vi "baseStation.vi"() -> ()   [LabVIEW 2012]
uses:
  <vilib>/Instr/_visa.llb/VISA Configure Serial Port (Instr).vi
panel:
  out "Cal Constants":u8[](array[numeric])
  in  "Auto Lock":bool
  in  "search mode":bool
  out "Found Radios":u8[](array[numeric])
  in  "shared variable refnum":refnum<k21>
  out "Humidity":dbl
  out "Temperature":dbl
  out "Pressure":dbl
  out "Magnetometer":dbl[](array[numeric])
  out "Gyro":dbl[](array[numeric])
  out "Acceleration":dbl[](array[numeric])
  out "Cal constants":string
  in  "State":T1(ring)
  out "output cluster":errorcluster
  in  "Stop Button":bool
  in  "Radio Address":dbl
  in  "Search for radio":bool
  in  "Com port":refnum<visa-resource-name>
  # "Active"
  # "Passive"
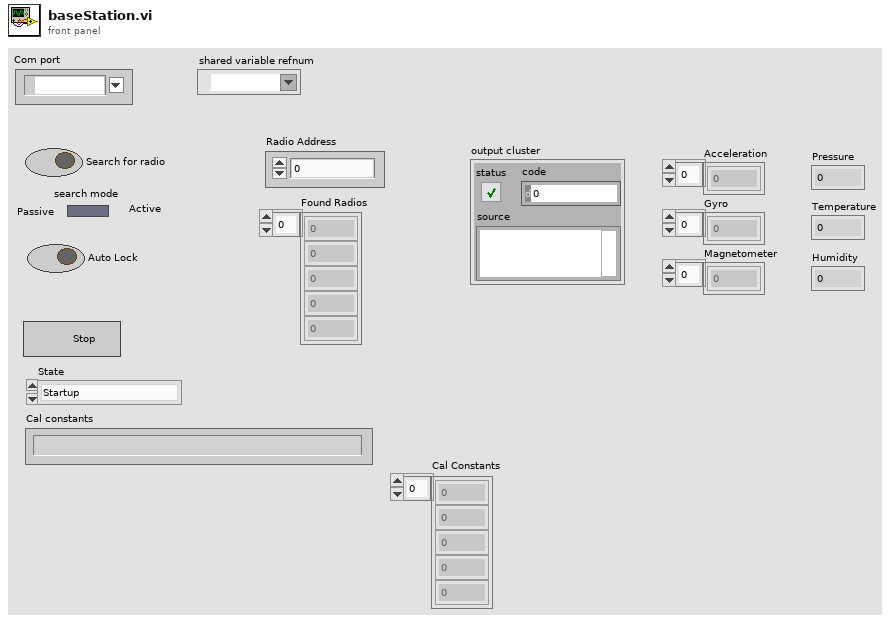
[diagram p1: front panel]
types:
  T1 = enum16{"Startup", "Start Search", "Active Search", "Start Single", "Run Single", "Shutdown", "Change Address"}
  T2 = cluster{"Acceleration":dbl[], "Gyro":dbl[], "Magnetometer":dbl[], "Temperature":dbl, "Pressure":dbl, "Humidity":dbl}
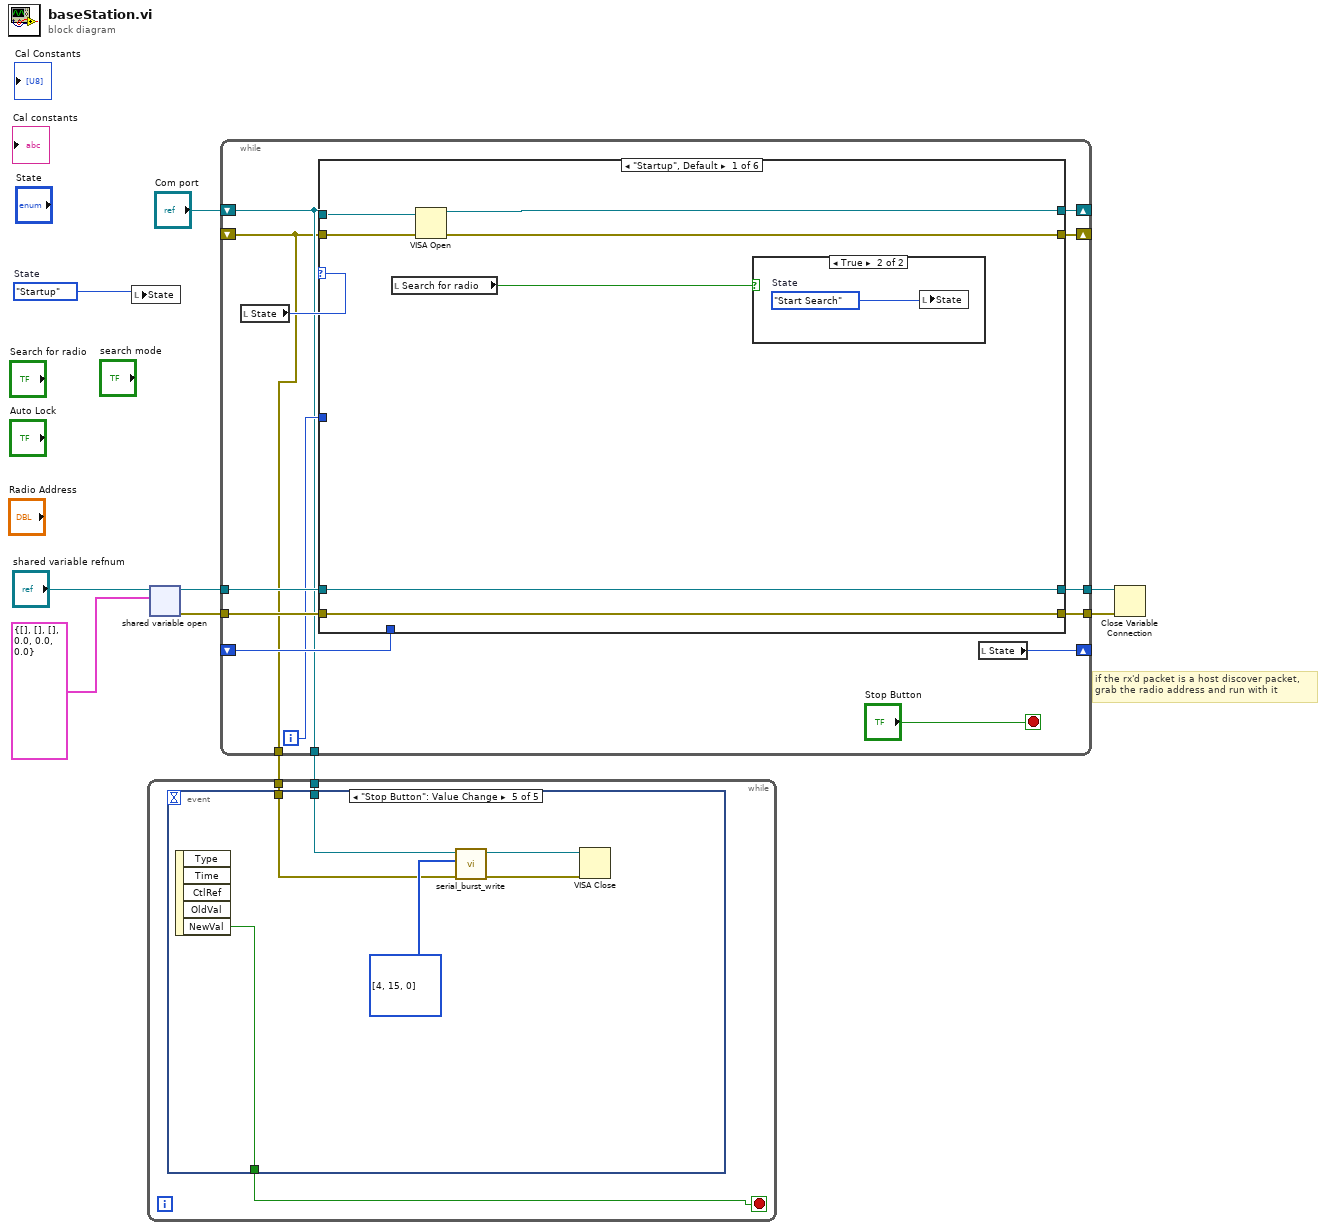
[diagram p0: block diagram]
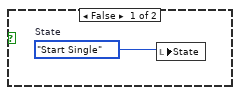
[diagram p2: hidden frame]
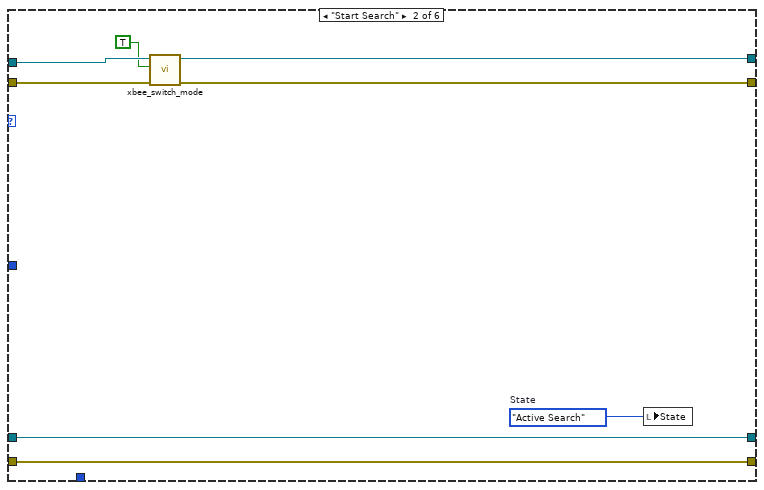
[diagram p3: hidden frame]
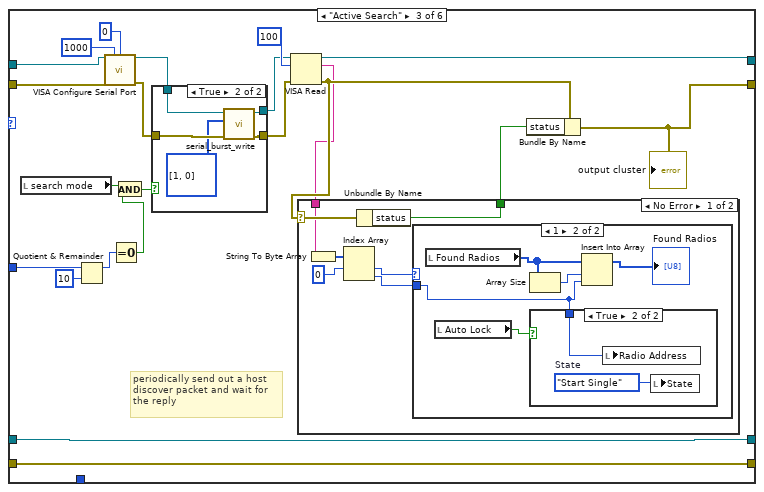
[diagram p4: hidden frame]
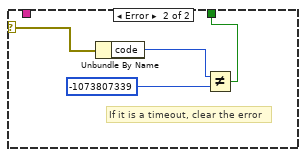
[diagram p8: hidden frame]
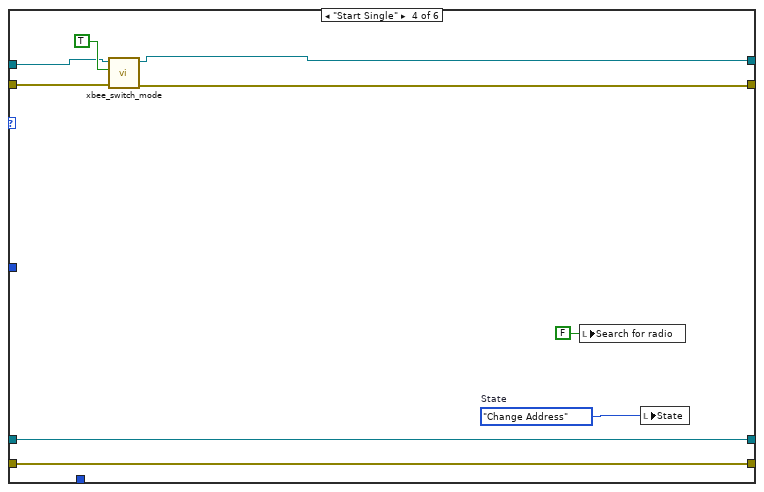
[diagram p9: hidden frame]
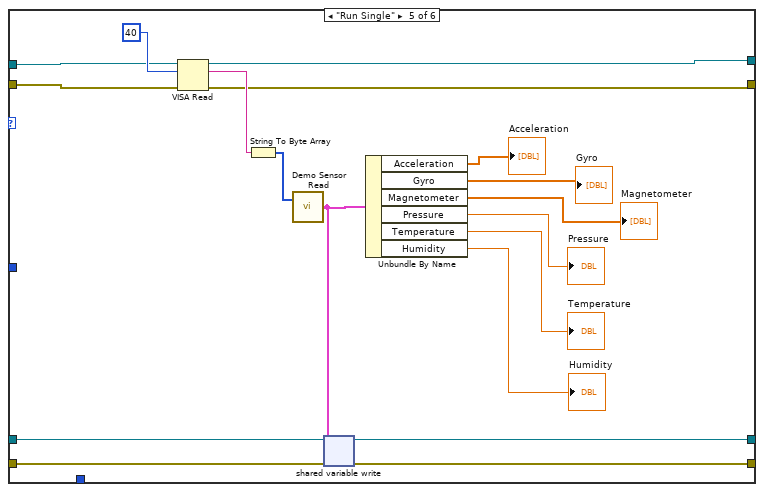
[diagram p10: hidden frame]
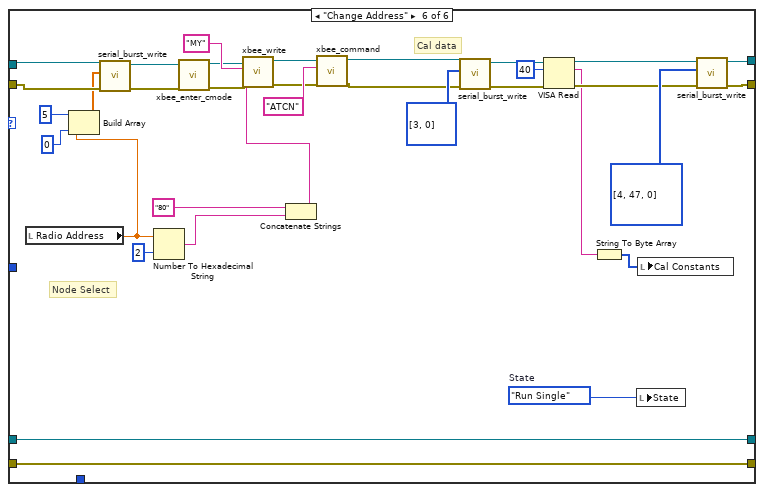
[diagram p11: hidden frame]
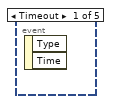
[diagram p12: hidden frame]
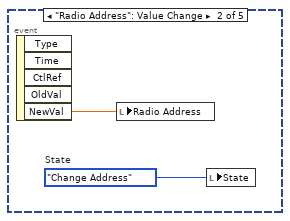
[diagram p13: hidden frame]
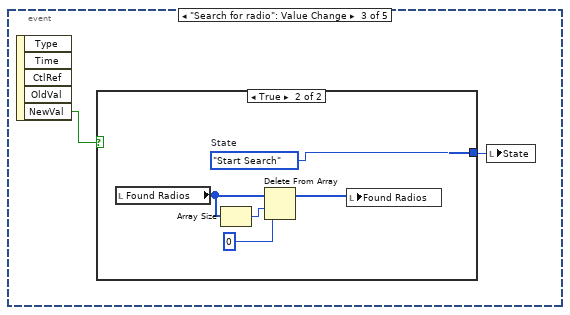
[diagram p14: hidden frame]
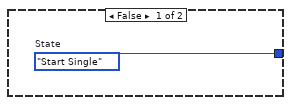
[diagram p15: hidden frame]
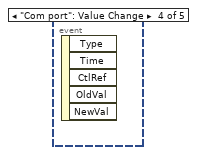
[diagram p16: hidden frame]
diagram:
  w3 = T1."Startup"  # State
  # "if the rx'd packet is a host discover packet,\ngrab the radio address and run with it"
  n1 = local write "State"(w3) -> ()
  n2 = shared-variable-open("shared variable refnum", T2 {"Acceleration"=[], "Gyro"=[], "Magnetometer"=[], "Temperature"=0.0, "Pressure"=0.0, "Humidity"=0.0} ("sensor output")) -> (w8:refnum<k21>, w7:errorcluster)  [unwired: 2 in]
  n3 = while {
    shift-right: [w23] -> _
    shift-left: "Com port" -> [w12]
    shift-right: [w22] -> _
    shift-left: _ -> [w11]
    tunnel: w8 -> [w19]
    tunnel: w7 -> [w18]
    tunnel: [w17] -> w6
    tunnel: [w16] -> w5
    shift-right: [w15] -> _
    shift-left: _ -> [w14]
    tunnel: [w12] -> w2
    tunnel: [w11] -> w1
    i -> [w13]
    stop <- "Stop Button" stop-if-true
    n4 = local read "State"() -> (w20:T1)
    n5 = case shown="\"Startup\", Default" w20 {
      tunnel: w12 -> [w30 w40 w59 w95 w112 w136]
      tunnel: [w28 w37 w58 w89 w110 w129] -> w23
      tunnel: [w27 w36 w57 w88 w109 w130] -> w22
      tunnel: w11 -> [w24 w39 w56 w94 w111 w135]
      tunnel: w19 -> [w26 w34 w52 w92 w101 w143]
      tunnel: w18 -> [w25 w33 w51 w91 w99 w142]
      tunnel: [w26 w34 w52 w92 w98 w143] -> w17
      tunnel: [w25 w33 w51 w91 w97 w142] -> w16
      tunnel: w14 -> [_ _ _ _ _ _]
      tunnel: w13 -> [_ _ w45 _ _ _]
      frame "Startup", Default {
        n6 = local read "Search for radio"() -> (w29:bool)
        n7 = VISA Open(error in (no error)=w24, VISA resource name=w30) -> (VISA resource name=w28:refnum<visa-resource-name>, error out=w27:errorcluster)  [unwired: 3 in]
        n8 = case shown="True" w29 {
          frame False {
            w31 = T1."Start Single"  # State
            n9 = local write "State"(w31) -> ()
          }
          frame True {
            w32 = T1."Start Search"  # State
            n10 = local write "State"(w32) -> ()
          }
        }
      }
      frame "Start Search" {
        w35 = T1."Active Search"  # State
        n11 = call "xbee_switch_mode.vi"("error in"=w39, "Global"=TRUE, "com in"=w40) -> ("error out"=w36:errorcluster, "com out"=w37:refnum<visa-resource-name>)  [unwired: 7 in]
        n12 = local write "State"(w35) -> ()
      }
      frame "Active Search" {
        # "periodically send out a host\ndiscover packet and wait for\nthe reply"
        n13 = local read "search mode"() -> (w42:bool)
        n14 = Quotient & Remainder(x=w45, y=10) -> (x-y*floor(x/y)=w46:i32)  [unwired: 1 out]
        n15 = call-poly "VISA Configure Serial Port"("VISA resource name"=w59, "timeout (10sec)"=u32 1000, "termination char\n(0xA = '\\n' = LF)"=u8 0 ("termination char\n(0xA = '\\n' = LF)"), "error in (no error)"=w56) -> ("VISA resource name out"=w50:refnum<visa-resource-name>, "error out"=w47:errorcluster)  [unwired: 10 in]
        n16 = Equal To 0?(x=w46) -> (x = 0?=w43:bool)
        n17 = And(x=w42, y=w43) -> (x .and. y?=w41:bool)
        n18 = case shown="True" w41 {
          tunnel: w50 -> [w64 w67]
          tunnel: [w64 w68] -> w49
          tunnel: [w63 w69] -> w48
          tunnel: w47 -> [w63 w66]
          frame False {
          }
          frame True {
            n19 = call "serial_burst_write.vi"("error in (no error)"=w66, "Byte array"=u16[] [1, 0], "VISA resource name"=w67) -> ("error out"=w69:errorcluster, "VISA resource name out"=w68:refnum<visa-resource-name>)  [unwired: 7 in]
          }
        }
        n20 = VISA Read(VISA resource name=w49, byte count=u32 100, error in (no error)=w48) -> (VISA resource name out=w58:refnum<visa-resource-name>, read buffer=w53:string, error out=w55:errorcluster)  [unwired: 1 out]
        n21 = case shown="No Error" w55 {
          selector: w55 -> [w76 w85]
          tunnel: [w75 w84] -> w54
          tunnel: w53 -> [w74 _]
          frame No Error {
            n22 = String To Byte Array(string=w74) -> (unsigned byte array=w73:u8[])
            n23 = Index Array(array=w73, index #1=0 ("index")) -> (element #1=w71:u8, element #2=w70:u8)  [unwired: 1 in]
            n24 = Unbundle By Name(w76) -> ("status"=w75:bool)
            n25 = case shown="1" w71 {
              tunnel: w70 -> [_ w77]
              frame 0, Default {
              }
              frame 1 {
                n26 = local read "Found Radios"() -> (w80:u8[])
                n27 = local read "Auto Lock"() -> (w78:bool)
                n28 = Array Size(array=w80) -> (size(s)=w81:i32)
                n29 = case shown="True" w78 {
                  tunnel: w77 -> [_ w82]
                  frame False {
                  }
                  frame True {
                    w83 = T1."Start Single"  # State
                    n30 = local write "Radio Address"(w82) -> ()
                    n31 = local write "State"(w83) -> ()
                  }
                }
                n32 = Insert Into Array(array=w80, index=w81, new element=w77) -> (→"Found Radios":u8[])
              }
            }
          }
          frame Error {
            # "If it is a timeout, clear the error"
            n33 = Unbundle By Name(w85) -> ("code"=w87:i32)
            n34 = Not Equal?(x=w87, y=-1073807339) -> (x != y?=w84:bool)
          }
        }
        n35 = Bundle By Name(cluster=w55, "status"=w54) -> (w57:errorcluster)
        "output cluster" <- w57
      }
      frame "Start Single" {
        w93 = T1."Change Address"  # State
        n36 = call "xbee_switch_mode.vi"("error in"=w94, "Global"=TRUE, "com in"=w95) -> ("error out"=w88:errorcluster, "com out"=w89:refnum<visa-resource-name>)  [unwired: 7 in]
        n37 = local write "Search for radio"(FALSE ("Search for radio")) -> ()
        n38 = local write "State"(w93) -> ()
      }
      frame "Run Single" {
        n39 = VISA Read(VISA resource name=w112, byte count=40, error in (no error)=w111) -> (VISA resource name out=w110:refnum<visa-resource-name>, read buffer=w114:string, error out=w109:errorcluster)  [unwired: 1 out]
        n40 = String To Byte Array(string=w114) -> (unsigned byte array=w108:u8[])
        n41 = call "Demo Sensor Read.vi"("Byte array"=w108) -> ("sensor output"=w100:T2)  [unwired: 1 in]
        n42 = shared-variable-write(w101, w99, w100) -> (w98:refnum<k21>, w97:errorcluster)
        n43 = Unbundle By Name(w100) -> ("Acceleration"=→"Acceleration":dbl[], "Gyro"=→"Gyro":dbl[], "Magnetometer"=→"Magnetometer":dbl[], "Pressure"=→"Pressure":dbl, "Temperature"=→"Temperature":dbl, "Humidity"=→"Humidity":dbl)
      }
      frame "Change Address" {
        w137 = T1."Run Single"  # State
        # "Cal data"
        # "Node Select"
        n44 = local read "Radio Address"() -> (w132:dbl)
        n45 = Build Array(u16 5 ("input string"), w132, 0 ("input string")) -> (w134:dbl[])
        n46 = call "serial_burst_write.vi"("error in (no error)"=w135, "Byte array"=w134, "VISA resource name"=w136) -> ("error out"=w122:errorcluster, "VISA resource name out"=w123:refnum<visa-resource-name>)  [unwired: 7 in]
        n47 = Number To Hexadecimal String(1:i16 2 ("width (-)"), 2:w132) -> (0:w147:string)
        n48 = call "xbee_enter_cmode.vi"("error in (no error)"=w122, "COM in"=w123) -> ("error out"=w120:errorcluster, "COM out"=w121:refnum<visa-resource-name>)  [unwired: 8 in]
        n49 = Concatenate Strings("80" ("string"), w147) -> (w145:string)
        n50 = call "xbee_write.vi"("error in"=w120, "value"=w145, "command"="MY", "com in"=w121) -> ("error out"=w116:errorcluster, "com out"=w118:refnum<visa-resource-name>)  [unwired: 6 in]
        n51 = call "xbee_command.vi"("error in (no error)"=w116, "command"="ATCN", "COM in"=w118) -> ("error out"=w115:errorcluster, "COM out"=w117:refnum<visa-resource-name>)  [unwired: 6 in, 1 out]
        n52 = call "serial_burst_write.vi"("error in (no error)"=w115, "Byte array"=u16[] [3, 0], "VISA resource name"=w117) -> ("error out"=w139:errorcluster, "VISA resource name out"=w140:refnum<visa-resource-name>)  [unwired: 7 in]
        n53 = VISA Read(VISA resource name=w140, byte count=u32 40, error in (no error)=w139) -> (VISA resource name out=w128:refnum<visa-resource-name>, read buffer=w125:string, error out=w126:errorcluster)  [unwired: 1 out]
        n54 = String To Byte Array(string=w125) -> (unsigned byte array=w124:u8[])
        n55 = local write "State"(w137) -> ()
        n56 = local write "Cal Constants"(w124) -> ()
        n57 = call "serial_burst_write.vi"("error in (no error)"=w126, "Byte array"=u16[] [4, 47, 0], "VISA resource name"=w128) -> ("error out"=w130:errorcluster, "VISA resource name out"=w129:refnum<visa-resource-name>)  [unwired: 7 in]
      }
    }
    n58 = local read "State"() -> (w15:T1)
  }
  n59 = while {
    tunnel: w2 -> [w150]
    tunnel: w1 -> [w149]
    stop <- w151 stop-if-true
    n60 = event shown="[4] \"Stop Button\": Value Change" {
      selector: _ -> [_ _ _ _ _]
      dyn-events: _ -> [_ _ _ _ _]
      timeout: _ -> [_ _ _ _ _]
      tunnel: [_ _ _ _ w167] -> w151
      tunnel: w150 -> [_ _ _ _ w165]
      tunnel: w149 -> [_ _ _ _ w164]
      event Timeout {
        n61 = event-data() -> ()  [unwired: 1 in, 2 out]
      }
      event "Radio Address": Value Change {
        w153 = T1."Change Address"  # State
        n62 = event-data() -> ("NewVal"=w152:dbl)  [unwired: 1 in, 4 out]
        n63 = local write "Radio Address"(w152) -> ()
        n64 = local write "State"(w153) -> ()
      }
      event "Search for radio": Value Change {
        n65 = event-data() -> ("NewVal"=w155:bool)  [unwired: 1 in, 4 out]
        n66 = case shown="True" w155 {
          tunnel: [w156 w161] -> w154
          frame False {
            w156 = T1."Start Single"  # State
          }
          frame True {
            w161 = T1."Start Search"  # State
            n67 = local read "Found Radios"() -> (w159:u8[])
            n68 = Array Size(array=w159) -> (size(s)=w160:i32)
            n69 = Delete From Array(array=w159, length=w160, index=0) -> (array with subset deleted=w158:u8[])  [unwired: 1 out]
            n70 = local write "Found Radios"(w158) -> ()
          }
        }
        n71 = local write "State"(w154) -> ()
      }
      event "Com port": Value Change {
        n72 = event-data() -> ()  [unwired: 1 in, 5 out]
      }
      event "Stop Button": Value Change {
        n73 = event-data() -> ("NewVal"=w167:bool)  [unwired: 1 in, 4 out]
        n74 = call "serial_burst_write.vi"("error in (no error)"=w164, "Byte array"=u16[] [4, 15, 0], "VISA resource name"=w165) -> ("error out"=w162:errorcluster, "VISA resource name out"=w163:refnum<visa-resource-name>)  [unwired: 7 in]
        n75 = VISA Close(VISA resource name=w163, error in (no error)=w162) -> ()  [unwired: 1 out]
      }
    }
  }
  n76 = Close Variable Connection(8:w5, 11:w6) -> ()  [unwired: 1 out]
